vi "Exit.vi"() -> (0 "Exit":bool)   [LabVIEW 2015]
uses:
  Galobal variable_TI.vi
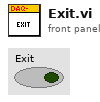
[diagram p1: front panel]
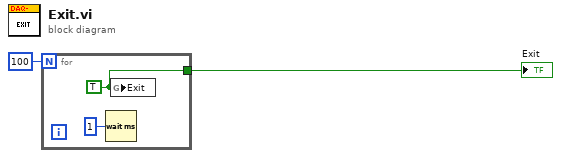
[diagram p0: block diagram]
diagram:
  n1 = for {
    N: 100 -> [_]
    tunnel: [w3] -> w2
    w3 = TRUE ("Exit")
    n2 = Wait (ms)(milliseconds to wait=u32 1) -> ()  [unwired: 1 out]
    n3 = global write "Galobal variable_TI.vi" "Exit"(w3) -> ()
  }
  "Exit" <- w2
